vi "Mode Reference.vi"(0 "INL DNL Test in":refnum<class "INL DNL Test.lvclass">, 11 "Error in":errorcluster) -> (4 "INL DNL Test out":refnum<class "INL DNL Test.lvclass">, 6 "VI Refnum":refnum<vi>, 15 "Error out":errorcluster)   [LabVIEW 2020, in "INL DNL Test.lvclass"]
doc: "Runs the mode page asynchronously."
uses:
  INL DNL Test.lvclass
  Parent/Typedef/LV2 Control.ctl
  Mode Page.vi
  Parent/Test.lvclass
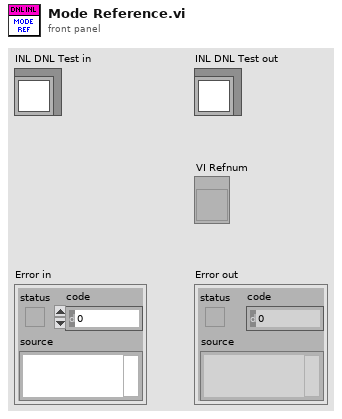
[diagram p1: front panel]
types:
  T1 = typedef "Test.lvclass/LV2 Control.ctl" = enum16{"Home", "Mode", "Config", "Status", "Read"}
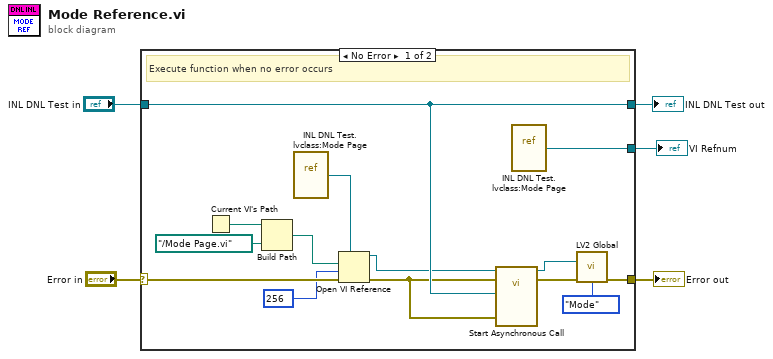
[diagram p0: block diagram]
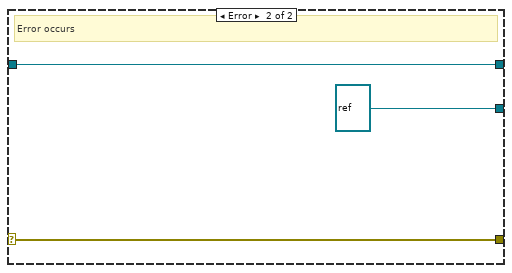
[diagram p2: hidden frame]
diagram:
  n1 = case shown="No Error" "Error in" {
    selector: "Error in" -> [w19 w21]
    tunnel: [w8 w21] -> w4
    tunnel: [w18 refnum<vi> refnum] -> w3
    tunnel: [w12 w22] -> w1
    tunnel: "INL DNL Test in" -> [w12 w22]
    frame No Error {
      # "Execute function when no error occurs"
      n2 = Current VI's Path() -> (path=w17:path)
      n3 = Build Path(base path=w17, name or relative path=path "../Mode Page.vi") -> (appended path=w15:path)
      n4 = vi-ref "INL DNL Test.lvclass:Mode Page.vi"() -> (w14:refnum<vi>)
      n5 = Open VI Reference(type specifier VI Refnum (for type only)=w14, vi path=w15, options=256, error in (no error)=w19) -> (vi reference=w9:refnum<vi>, error out=w11:errorcluster)  [unwired: 2 in]
      n6 = call-by-ref "Start Asynchronous Call"(reference=w9, error in=w11, "Error in"=w11, "reference out 2"=w12) -> (reference out=w6:refnum<vi>, error out=w10:errorcluster)  [unwired: 8 in, 2 out]
      n7 = vi-ref "INL DNL Test.lvclass:Mode Page.vi"() -> (w18:refnum<vi>)
      n8 = call "LV2 Global.vi"("Mode Ref In"=w6, "Error In"=w10, "Enum"=LV2_Control."Mode") -> ("Error Out"=w8:errorcluster)  [unwired: 8 in, 4 out]
    }
    frame Error {
      # "Error occurs"
    }
  }
  "Error out" <- w4
  "INL DNL Test out" <- w1
  "VI Refnum" <- w3
